vi "DisconnectFromRobot.vi"(0 "error in":errorcluster, 4 "robot":refnum<k24>) -> (20 "error out":errorcluster)   [LabVIEW 2012, in "UnderAutomation.Fanuc.lvlib"]
uses:
  UnderAutomation.Fanuc.lvlib
  C:/Users/fg/Documents/Fanuc.vi/LabVIEW_2024/UnderAutomation.Fanuc/lib/UnderAutomation.Fanuc.dll
  LabVIEW_2024/UnderAutomation.Fanuc/lib/UnderAutomation.Fanuc.dll
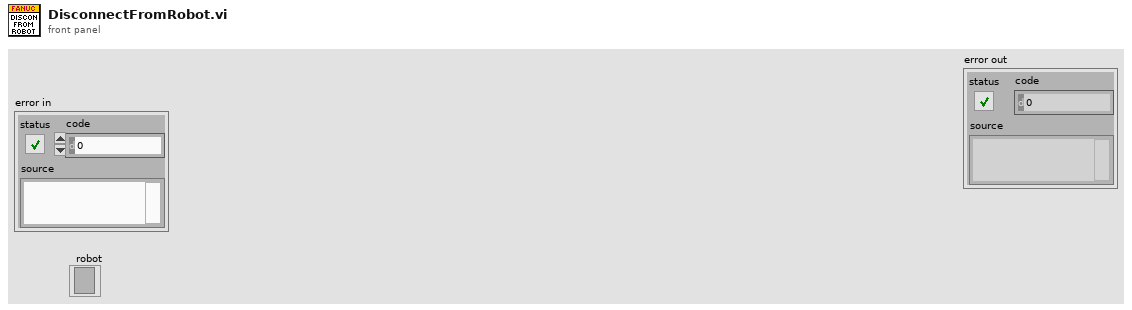
[diagram p1: front panel]
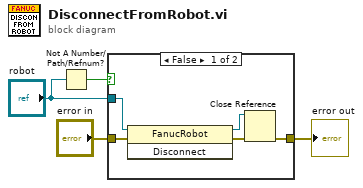
[diagram p0: block diagram]
diagram:
  n1 = Not A Number/Path/Refnum?(number/path/refnum="robot") -> (NaN/Path/Refnum?=w4:bool)
  n2 = case shown="False" w4 {
    tunnel: "robot" -> [w9 _]
    tunnel: "error in" -> [w8 w10]
    tunnel: [w5 w10] -> w1
    frame False {
      n3 = invoke class="FanucRobot" method="Disconnect"(reference=w9, error in=w8) -> (reference out=w6:refnum<k24>, error out=w7:errorcluster)  [unwired: 1 in, 1 out]
      n4 = Close Reference(reference=w6, error in (no error)=w7) -> (error out=w5:errorcluster)
    }
    frame True {
    }
  }
  "error out" <- w1
